vi "A(SubVI).vi"(8 "Lambda":dbl[](array[numeric]), 9 "I(blank)":dbl[](array[numeric]), 10 "I(dark)":dbl[](array[numeric]), 11 "I":dbl[](array[numeric])) -> (3 "Aout":dbl[](array[numeric]))   [LabVIEW 2019]
uses:
  Global.vi
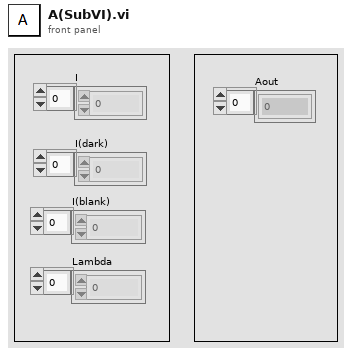
[diagram p1: front panel]
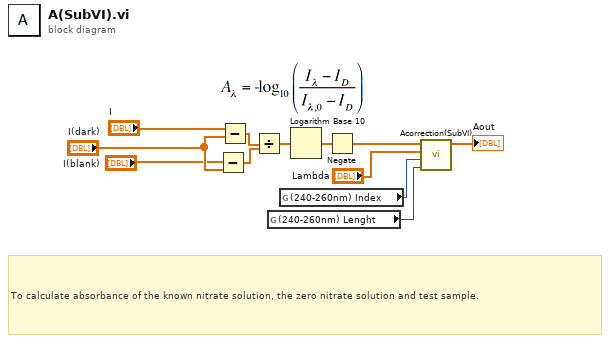
[diagram p0: block diagram]
diagram:
  # "To calculate absorbance of the known nitrate solution, the zero nitrate solution and test sample."
  n1 = Subtract(x="I(blank)", y="I(dark)") -> (x-y=w6:dbl[])
  n2 = Subtract(x="I", y="I(dark)") -> (x-y=w5:dbl[])
  n3 = Divide(x=w5, y=w6) -> (x/y=w7:dbl[])
  n4 = global read "Global.vi" "(240-260nm) Lenght"() -> (w3:i32)
  n5 = global read "Global.vi" "(240-260nm) Index"() -> (w4:i32)
  n6 = Logarithm Base 10(1:w7) -> (0:w8:dbl[])
  n7 = Negate(x=w8) -> (-x=w9:dbl[])
  n8 = call "Acorrection(SubVI).vi"("length"=w3, "index"=w4, "Lambda"="Lambda", "Ain"=w9) -> ("Aout"=→"Aout":dbl[])  [unwired: 6 in, 1 out]
